vi "Read Configuration File.vi"(8 "error in (no error)":errorcluster, 11 "Instrument.KH7008 in":refnum<class "Instrument.KH7008.lvclass">) -> (0 "error out":errorcluster, 3 "Instrument.KH7008 out":refnum<class "Instrument.KH7008.lvclass">)   [LabVIEW 2019, in "Instrument.KH7008.lvclass"]
uses:
  Instrument.KH7008.lvclass
  <userlib>/LevyLab/Levylab Instruments/SMOs/Instrument/Instrument.lvclass
  <userlib>/LevyLab/Levylab Instruments/SMOs/Configuration/Configuration.lvclass
  C:/Program Files (x86)/National Instruments/LabVIEW 2019/user.lib/LevyLab/Levylab Instruments/SMOs/Instrument/Instrument.lvclass
  C:/Program Files (x86)/National Instruments/LabVIEW 2019/vi.lib/JKI/JKI SMO/SMO/SMO.lvclass
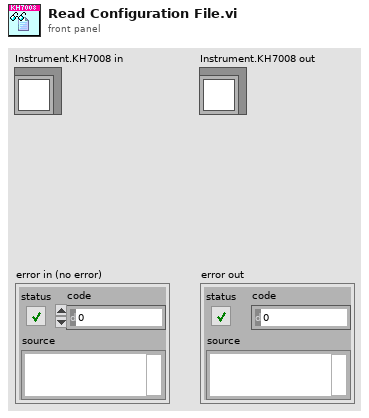
[diagram p1: front panel]
types:
  T1 = typedef "Instrument.KH7008.lvclass/SetAll-Array.ctl" = T2[]
  T2 = typedef "Instrument.KH7008.lvclass/SetAll-Cluster.ctl" = cluster{"Channel":T3, "Gain":T4, "Bandwidth Filter":T5, "Shunt Resistor":T6, "Coupling":T7, "Input Config":T8}
  T3 = typedef "Instrument.KH7008.lvclass/Channel-Enum.ctl" = enum16{"Channel 1", "Channel 2", "Channel 3", "Channel 4", "Channel 5", "Channel 6", "Channel 7", "Channel 8"}
  T4 = typedef "Instrument.KH7008.lvclass/Gain-Enum.ctl" = enum16{"1x", "10x", "100x", "1000x"}
  T5 = typedef "Instrument.KH7008.lvclass/Filter-Enum.ctl" = enum16{"OFF", "ON"}
  T6 = typedef "Instrument.KH7008.lvclass/Shunt-Enum.ctl" = enum16{"Open", "50 Ohms", "500 Ohms", "5k Ohms", "50k Ohms", "10M Ohm"}
  T7 = typedef "Instrument.KH7008.lvclass/Coupling-Enum.ctl" = enum16{"AC", "DC"}
  T8 = typedef "Instrument.KH7008.lvclass/Input Configuration-Enum.ctl" = enum16{"Ground", "SE+ (-gnd)", "SE- (+gnd)", "Differential"}
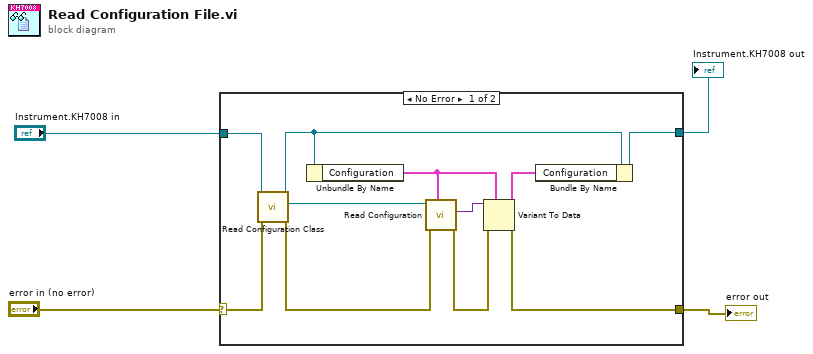
[diagram p0: block diagram]
diagram:
  n1 = case shown="No Error" "error in (no error)" {
    selector: "error in (no error)" -> [w12 w17]
    tunnel: [w11 w17] -> w3
    tunnel: [w15 w16] -> w1
    tunnel: "Instrument.KH7008 in" -> [w14 w16]
    frame No Error {
      n2 = call <userlib>:"Read Configuration Class.vi"("error in (no error)"=w12, "Instrument in"=w14) -> ("error out"=w9:errorcluster, "Configuration"=w8:refnum<class "Configuration.lvclass">, "Instrument out"=w13:refnum<class "Instrument.KH7008.lvclass">)  [unwired: 7 in]
      n3 = Unbundle By Name(w13) -> ("Configuration"=w10:cluster{"Channel Setting":T1, "Gain":dbl[]})
      n4 = call <userlib>:"Read Configuration.vi"("INI Fomatted Cluster Type"=w10, "error in (no error)"=w9, "Configuration in"=w8) -> ("error out"=w6:errorcluster, "Configuration"=w7:variant)  [unwired: 6 in, 1 out]
      n5 = Variant To Data(error in=w6, type=w10, Variant=w7) -> (data=w5:cluster{"Channel Setting":T1, "Gain":dbl[]}, error out=w11:errorcluster)
      n6 = Bundle By Name(cluster=w13, "Configuration"=w5) -> (w15:refnum<class "Instrument.KH7008.lvclass">)
    }
    frame Error {
    }
  }
  "Instrument.KH7008 out" <- w1
  "error out" <- w3
